vi "frontPanel.vi"(8 "error in (no error)":errorcluster, 10 "closeViewerEvent":refnum<user-event>, 11 "FringeTestingViewer in":refnum<class "FringeTestingViewer.lvclass">) -> (0 "error out":errorcluster, 3 "FringeTestingViewer out":refnum<class "FringeTestingViewer.lvclass">)   [LabVIEW 2011, in "Views.lvlib" / "Camera.lvlib" / "FringeTestingViewer.lvclass"]
uses:
  FringeTestingViewer.lvclass
  Tools/Filing/FileNeologist/FileNeologist.lvclass
panel:
  out "Numeric":dbl format="%^#.6g"
  in  "stop":bool
  out "XY Graph":cluster{dbl[], dbl[]}(graph)
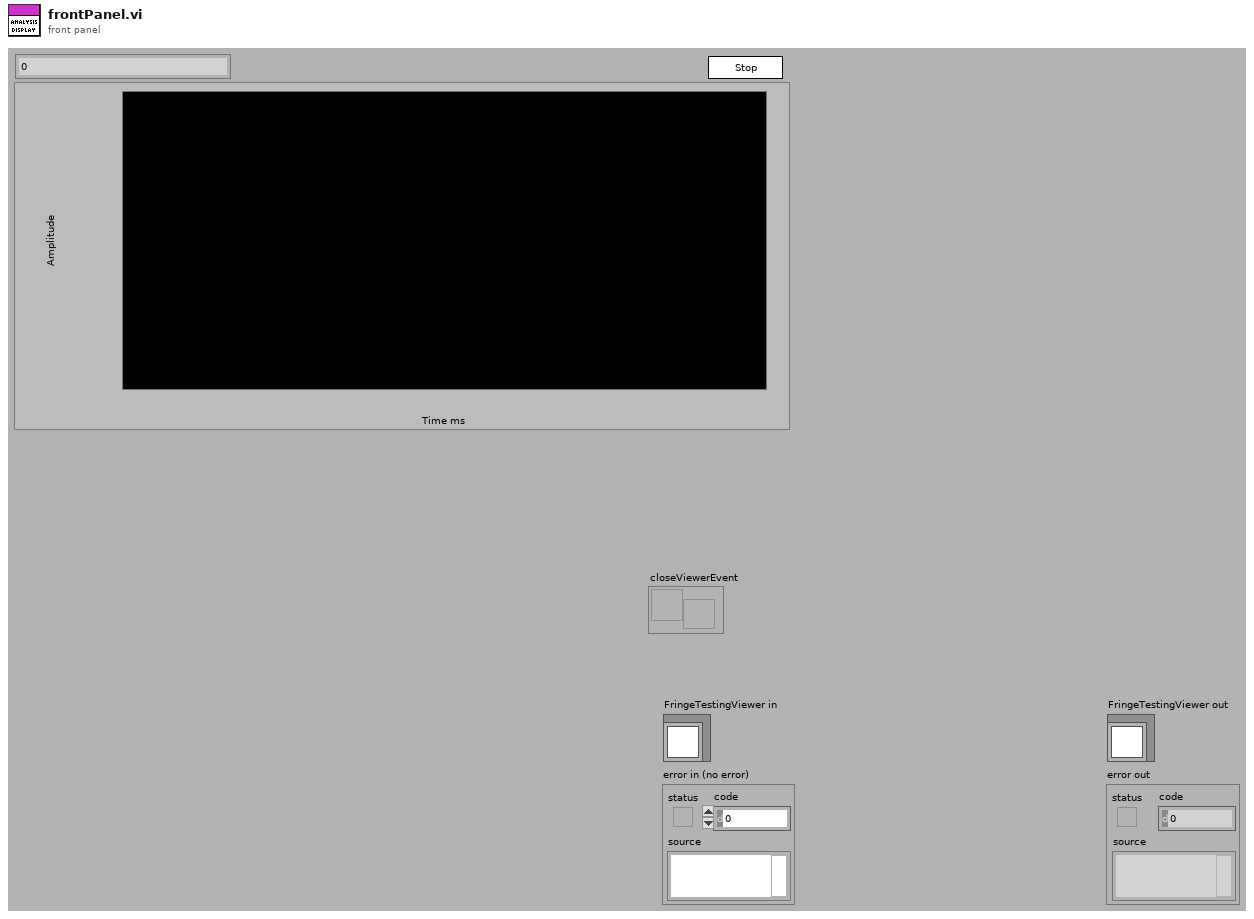
[diagram p1: front panel]
types:
  T1 = cluster{"Name":string, "Results":dbl[], "AnalysisType":string}
  T2 = enum16{"open", "replace", "create", "open or create", "replace or create", "replace or create with confirmation"}
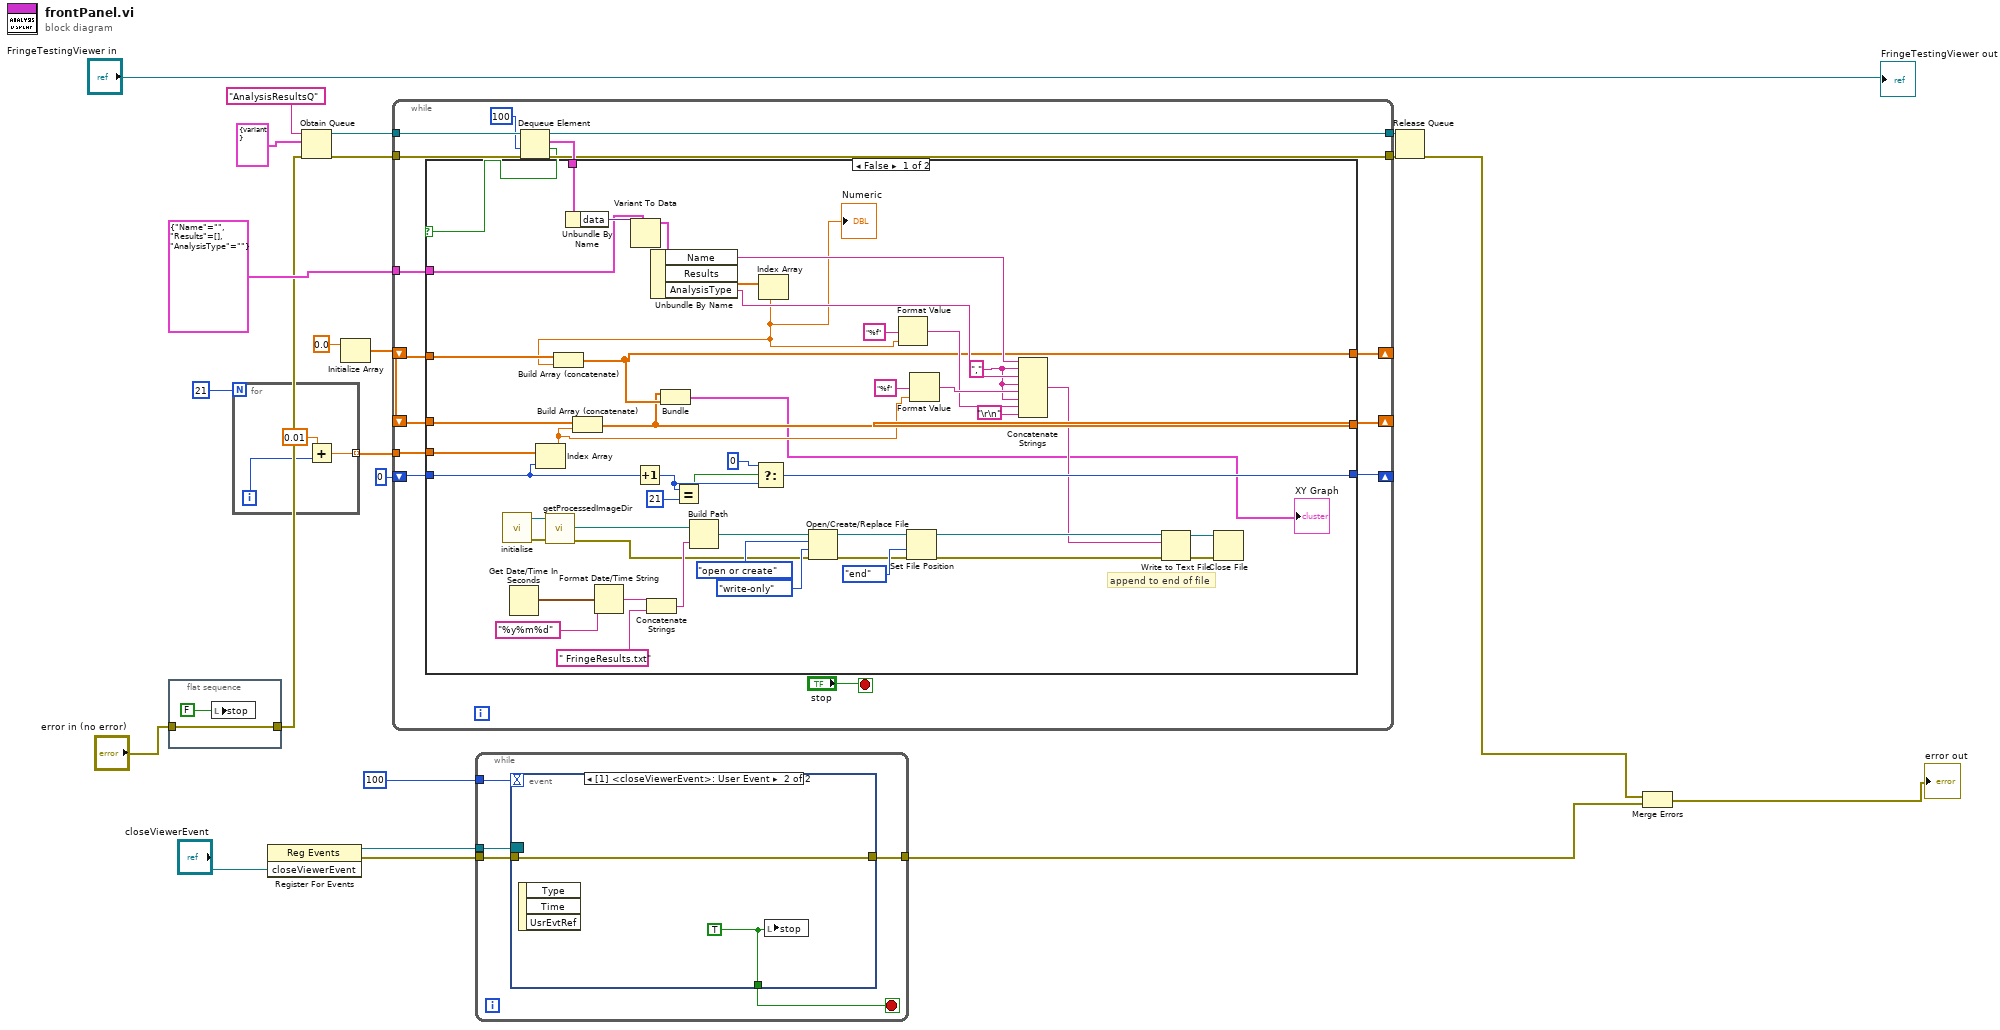
[diagram p0: block diagram]
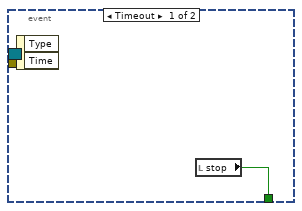
[diagram p2: hidden frame]
diagram:
  n1 = flat-sequence {
    tunnel: "error in (no error)" -> [w24]
    tunnel: [w24] -> w3
    frame #0 {
      n2 = local write "stop"(FALSE) -> ()
    }
  }
  n3 = for {
    N: 21 -> [_]
    tunnel: [w25] -> w16 mode=indexing
    i -> [w26]
    n4 = Add(x=0.01, y=w26) -> (x+y=w25:dbl)
  }
  n5 = register-events("closeViewerEvent") -> (reference out=w10:refnum<event-registration>, error out=w8:errorcluster)  [unwired: 2 in]
  n6 = Obtain Queue(name (unnamed)="AnalysisResultsQ", element data type=cluster{"data":variant} {"data"=variant} ("dataQ"), error in (no error)=w3) -> (queue out=w21:refnum<queue>, error out=w20:errorcluster)  [unwired: 2 in, 1 out]
  n7 = Initialize Array(0.0) -> (w1:dbl[])  [unwired: 1 in]
  n8 = while {
    tunnel: w21 -> [w35]
    tunnel: w20 -> [w34]
    tunnel: T1 {"Name"="", "Results"=[], "AnalysisType"=""} ("output cluster") -> [w32]
    tunnel: w16 -> [w42]
    shift-right: [w40] -> _
    shift-left: w1 -> [w41]
    shift-right: [w39] -> _
    shift-left: w1 -> [w38]
    shift-right: [w36] -> _
    shift-left: 0 -> [w37]
    tunnel: [w31] -> w14
    tunnel: [w30] -> w13
    stop <- "stop" stop-if-true
    n9 = Dequeue Element(queue=w35, timeout in ms (-1)=100, error in (no error)=w34) -> (queue out=w31:refnum<queue>, element=w33:cluster{"data":variant}, timed out?=w28:bool, error out=w30:errorcluster)
    n10 = case shown="False" w28 {
      tunnel: w42 -> [w90 _]
      tunnel: w41 -> [w89 w92]
      tunnel: [w47 w92] -> w40
      tunnel: [w48 w93] -> w39
      tunnel: w38 -> [w88 w93]
      tunnel: w37 -> [w87 w91]
      tunnel: [w86 w91] -> w36
      tunnel: w33 -> [w82 _]
      tunnel: w32 -> [w79 _]
      frame False {
        w52 = ","
        # "append to end of file"
        n11 = call "initialise.vi"() -> ("error out"=w76:errorcluster, "FileNeologist out"=w77:refnum<class "FileNeologist.lvclass">)  [unwired: 10 in]
        n12 = Get Date/Time In Seconds() -> (seconds since 1Jan1904=w74:timestamp)
        n13 = Index Array(array=w90, index=w87) -> (element=w57:dbl)
        n14 = call-dynamic "getProcessedImageDir.vi"("error in (no error)"=w76, "FileNeologist in"=w77) -> ("error out"=w65:errorcluster, "Path"=w75:path)  [unwired: 7 in, 1 out]
        n15 = Unbundle By Name(w82) -> ("data"=w81:variant)
        n16 = Build Array (concatenate)(w89, w57) -> (w47:dbl[])
        n17 = Format Date/Time String(time format string (%c)="%y%m%d", seconds (now)=w74) -> (date/time string=w72:string)  [unwired: 1 in]
        n18 = Variant To Data(type=w79, Variant=w81) -> (data=w80:T1)  [unwired: 1 in, 1 out]
        n19 = Increment(x=w87) -> (x+1=w85:i32)
        n20 = Concatenate Strings(w72, " FringeResults.txt") -> (w70:string)
        n21 = Unbundle By Name(w80) -> ("Name"=w55:string, "Results"=w78:dbl[], "AnalysisType"=w54:string)
        n22 = Equal?(x=w85, y=21) -> (x = y?=w46:bool)
        n23 = Build Path(base path=w75, name or relative path=w70) -> (appended path=w69:path)
        n24 = Select(t=0, s=w46, f=w85) -> (s? t:f=w86:i32)
        n25 = Index Array(array=w78) -> (element=w44:dbl)  [unwired: 1 in]
        "Numeric" <- w44
        n26 = Build Array (concatenate)(w88, w44) -> (w48:dbl[])
        n27 = Bundle(w47, w48) -> (→"XY Graph":cluster{dbl[], dbl[]})  [unwired: 1 in]
        n28 = Open/Create/Replace File(file path (use dialog)=w69, error in=w65, operation (0:open)=T2."open or create", access (0:read/write)=enum16{"read/write", "read-only", "write-only"}."write-only") -> (refnum out=w68:refnum<file>, error out=w60:errorcluster)  [unwired: 2 in, 1 out]
        n29 = Format Value(format string="%f", value (0)=w44) -> (output string=w51:string)  [unwired: 1 in]
        n30 = Set File Position(refnum=w68, from (0:start)=enum16{"start", "end", "current"}."end", error in=w60) -> (refnum out=w62:refnum<file>, error out=w59:errorcluster)  [unwired: 1 in]
        n31 = Format Value(format string="%f", value (0)=w57) -> (output string=w53:string)  [unwired: 1 in]
        n32 = Concatenate Strings(w55, w52, w54, w52, w53, w52, w51, "\r\n") -> (w49:string)
        n33 = Write to Text File(file (use dialog)=w62, text=w49, error in=w59) -> (refnum out=w63:refnum<file>, error out=w64:errorcluster)  [unwired: 1 in, 1 out]
        n34 = Close File(refnum=w63, error in=w64) -> ()  [unwired: 2 out]
      }
      frame True {
      }
    }
  }
  n35 = while {
    tunnel: w10 -> [w98]
    tunnel: 100 -> [w96]
    tunnel: w8 -> [w95]
    tunnel: [w94] -> w7
    stop <- w97 stop-if-true
    n36 = event shown="[1] <closeViewerEvent>: User Event" {
      selector: w98 -> [_ _]
      dyn-events: _ -> [_ _]
      timeout: w96 -> [_ _]
      tunnel: [w99 w101] -> w97
      tunnel: w95 -> [_ w100]
      tunnel: [_ w100] -> w94
      event Timeout {
        n37 = event-data() -> ()  [unwired: 1 in, 2 out]
        n38 = local read "stop"() -> (w99:bool)
      }
      event User Event {
        w101 = TRUE
        n39 = event-data() -> ()  [unwired: 1 in, 3 out]
        n40 = local write "stop"(w101) -> ()
      }
    }
  }
  n41 = Release Queue(queue=w14, error in (no error)=w13) -> (error out=w6:errorcluster)  [unwired: 1 in, 2 out]
  n42 = Merge Errors(w6, w7) -> (→"error out":errorcluster)
  "FringeTestingViewer out" <- "FringeTestingViewer in"
